vi "Decode FST200 Speed Response.vi"(10 "Modbus Response":string) -> (1 "Frame Valid?":bool, 2 "Wind Speed (m/s)":dbl)   [LabVIEW 2026]
panel:
  out "CRC Valid?":bool
  out "Received CRC":u16
  out "Basic Frame Valid??":bool
  out "Raw Speed Register":u16
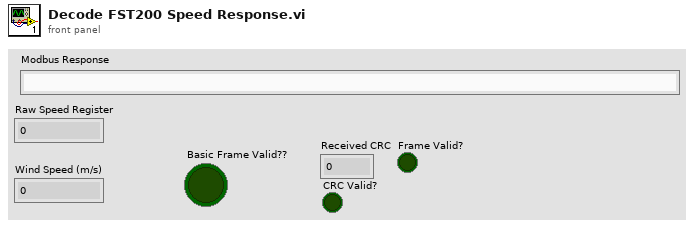
[diagram p1: front panel]
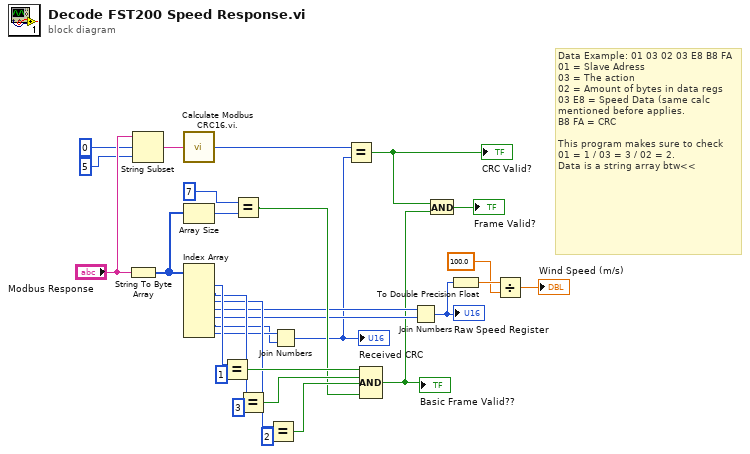
[diagram p0: block diagram]
diagram:
  # "Data Example: 01 03 02 03 E8 B8 FA\n01 = Slave Adress\n03 = The action\n02 = Amount of bytes in data regs\n03 E8 = Speed Data (same calc mentioned before applies.\nB8 FA = CRC\n\nThis program makes sure to check\n01 = 1 / 03 = 3 / 02 = 2.\nData is a string array btw<<"
  n1 = String To Byte Array(string="Modbus Response") -> (unsigned byte array=w26:u8[])
  n2 = String Subset(string="Modbus Response", offset (0)=0, length (rest)=5 ("length (rest)")) -> (substring=w8:string)
  n3 = call "Calculate Modbus CRC16.vi..vi"("Data Bytes"=w8) -> ("Calculated CRC"=w4:u16)
  n4 = Array Size(array=w26) -> (size(s)=w25:i32)
  n5 = Index Array(array=w26) -> (element #1=w23:u8, element #2=w21:u8, element #3=w14:u8, element #4=w13:u8, element #5=w12:u8, element #6=w6:u8, element #7=w7:u8)  [unwired: 7 in]
  n6 = Equal?(x=w23, y=u8 1) -> (x = y?=w18:bool)
  n7 = Equal?(x=7, y=w25) -> (x = y?=w15:bool)
  n8 = Equal?(x=w21, y=u8 3) -> (x = y?=w17:bool)
  n9 = Equal?(x=w14, y=u8 2) -> (x = y?=w16:bool)
  n10 = Join Numbers(hi=w7, lo=w6) -> ((hi.lo)=w5:u16)
  "Received CRC" <- w5
  n11 = Equal?(x=w4, y=w5) -> (x = y?=w3:bool)
  "CRC Valid?" <- w3
  n12 = Compound Arithmetic op=AND(w18, w17, w16, w15) -> (w2:bool)
  "Basic Frame Valid??" <- w2
  n13 = Join Numbers(hi=w13, lo=w12) -> ((hi.lo)=w30:u16)
  "Raw Speed Register" <- w30
  n14 = And(x=w3, y=w2) -> (x .and. y?=→"Frame Valid?":bool)
  n15 = To Double Precision Float(number=w30) -> (double precision float=w29:dbl)
  n16 = Divide(x=w29, y=100.0) -> (x/y=→"Wind Speed (m/s)":dbl)
